vi "NtfyLvFpga_SUB_ReadResultFromLogfile.vi"(8 "エラー入力":errorcluster, 11 "filepath":path=path "lvXilinxLog.txt") -> (0 "エラー出力":errorcluster, 2 "UTF8 TEXT":string)   [LabVIEW 2013]
panel:
  out "長さ":i32
  out "SJIS TEXT":string
  # "ログ・ファイル末尾の結果１０行分だけ読み込み"
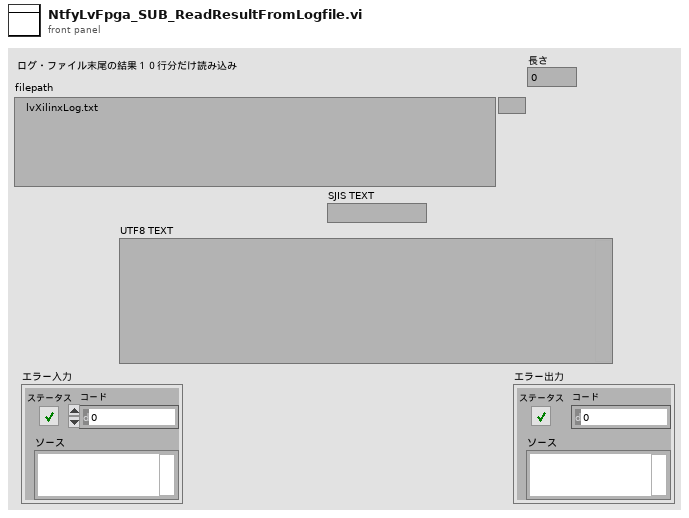
[diagram p1: front panel]
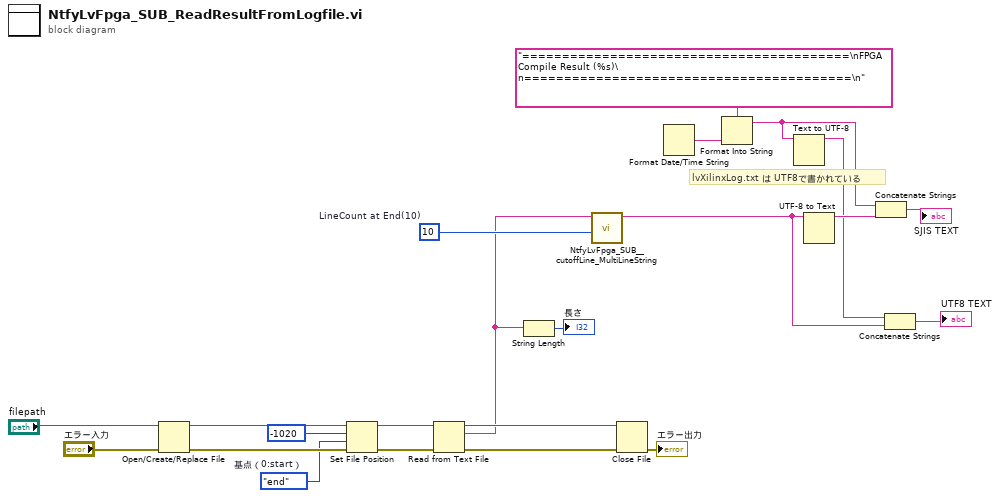
[diagram p0: block diagram]
diagram:
  w12 = enum16{"start", "end", "current"}."end"  # 基点（0:start）
  w20 = 10  # LineCount at End(10)
  # "lvXilinxLog.txt は UTF8で書かれている"
  n1 = Open/Create/Replace File(file path (use dialog)="filepath", error in="エラー入力") -> (refnum out=w14:refnum<file>, error out=w13:errorcluster)  [unwired: 4 in, 1 out]
  n2 = Set File Position(offset (in bytes) (0)=i64 -1020, refnum=w14, from (0:start)=w12, error in=w13) -> (refnum out=w16:refnum<file>, error out=w15:errorcluster)
  n3 = Read from Text File(file (use dialog)=w16, error in=w15) -> (refnum out=w18:refnum<file>, text=w10:string, error out=w17:errorcluster)  [unwired: 2 in, 1 out]
  n4 = String Length(string=w10) -> (length=→"長さ":i32)
  n5 = call "NtfyLvFpga_SUB__cutoffLine_MultiLineString.vi"("LineCount at End(1000)"=w20, "String"=w10) -> ("String out"=w5:string)  [unwired: 9 in]
  n6 = Close File(refnum=w18, error in=w17) -> (error out=→"エラー出力":errorcluster)  [unwired: 1 out]
  n7 = Format Date/Time String() -> (date/time string=w3:string)  [unwired: 3 in]
  n8 = Format Into String(format string="=========================================\nFPGA Compile Result (%s)\n=========================================\n", w3) -> (resulting string=w2:string)  [unwired: 2 in, 1 out]
  n9 = Text to UTF-8(11:w2) -> (3:w6:string)  [unwired: 1 in, 1 out]
  n10 = UTF-8 to Text(11:w5) -> (3:w8:string)  [unwired: 1 in, 1 out]
  n11 = Concatenate Strings(w2, w8) -> (→"SJIS TEXT":string)
  n12 = Concatenate Strings(w6, w5) -> (→"UTF8 TEXT":string)
